vi "LoadMasks.vi"(10 "UiDefinition 2":T1, 11 "ComboBox in":refnum<vi>) -> (0 "error out":errorcluster)   [LabVIEW 2020]
uses:
  UIReferences.ctl
  D:/LabviewDXFViewer/LabviewDXFViewer/bin/Release/LabviewDXFViewer.exe
  LabviewDXFViewer/bin/Release/LabviewDXFViewer.exe
  <vilib>/httpClient/LabVIEWHTTPClient.lvlib
panel:
  out "Array":errorcluster[](array[cluster])
  out "error out 2":errorcluster
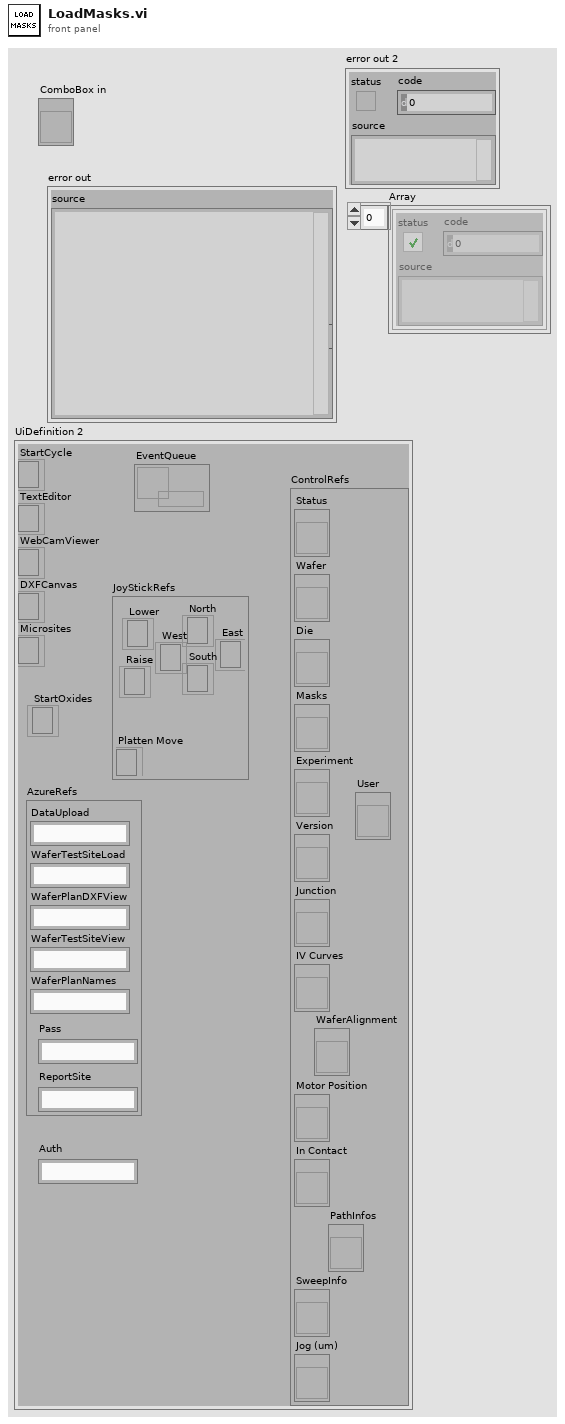
[diagram p1: front panel]
types:
  T1 = typedef "UIReferences.ctl" = cluster{"StartCycle":refnum<k24>, "TextEditor":refnum<k24>, "WebCamViewer":refnum<k24>, "DXFCanvas":refnum<k24>, "Microsites":refnum<k24>, "JoyStickRefs":cluster{"North":refnum<k24>, "Lower":refnum<k24>, "Raise":refnum<k24>, "Platten Move":refnum<k24>, "West":refnum<k24>, "East":refnum<k24>, "South":refnum<k24>}, "AzureRefs":cluster{"DataUpload":string, "WaferTestSiteLoad":string, "WaferPlanDXFView":string, "WaferTestSiteView":string, "WaferPlanNames":string, "Pass":string, "ReportSite":string}, "ControlRefs":cluster{"Status":refnum<vi>, "Wafer":refnum<vi>, "Die":refnum<vi>, "Masks":refnum<vi>, "Experiment":refnum<vi>, "Version":refnum<vi>, "Junction":refnum<vi>, "IV Curves":refnum<vi>, "Motor Position":refnum<vi>, "In Contact":refnum<vi>, "SweepInfo":refnum<vi>, "Jog (um)":refnum<vi>, "PathInfos":refnum<vi>, "User":refnum<vi>, "WaferAlignment":refnum<vi>}, "EventQueue":refnum<queue>, "StartOxides":refnum<k24>, "Auth":string}
  T2 = typedef "LabVIEWHTTPClient.lvlib/ClientHandle.ctl" = refnum<k1>
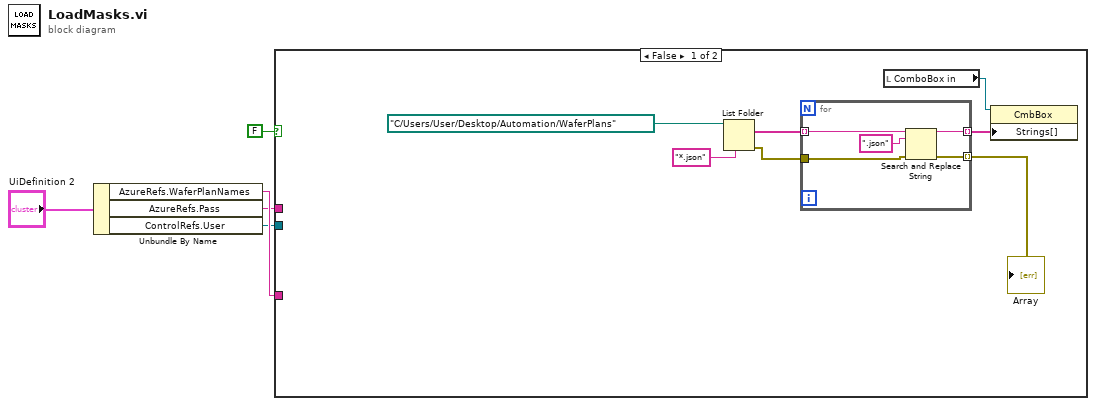
[diagram p0: block diagram]
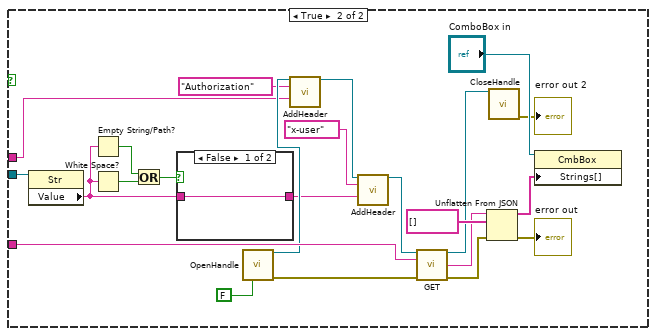
[diagram p2: hidden frame]
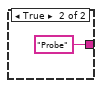
[diagram p3: hidden frame]
diagram:
  n1 = Unbundle By Name("UiDefinition 2") -> ("AzureRefs.WaferPlanNames"=w4:string, "AzureRefs.Pass"=w3:string, "ControlRefs.User"=w2:refnum<vi>)
  n2 = case shown="False" FALSE {
    tunnel: w4 -> [_ w32]
    tunnel: w3 -> [_ w27]
    tunnel: w2 -> [_ w25]
    frame False {
      n3 = List Folder(path=path "C:/Users/User/Desktop/Automation/WaferPlans", pattern="*.json") -> (filenames=w9:string[], error out=w7:errorcluster)  [unwired: 2 in, 2 out]
      n4 = for {
        tunnel: w9 -> [w17] mode=indexing
        tunnel: [w15] -> w8 mode=indexing
        tunnel: w7 -> [w14]
        tunnel: [w13] -> w6 mode=indexing
        n5 = Search and Replace String(input string=w17, search string=".json" ("substring (\"\")"), error in=w14) -> (result string=w15:string, error out=w13:errorcluster)  [unwired: 5 in, 2 out]
      }
      "Array" <- w6
      n6 = local read "ComboBox in"() -> (w11:refnum<vi>)
      n7 = property class="CmbBox"(reference=w11, "Strings[]"=w8) -> ()  [unwired: 1 in, 2 out]
    }
    frame True {
      n8 = property class="Str"(reference=w25) -> ("Value"=w20:string)  [unwired: 1 in, 2 out]
      n9 = Empty String/Path?(string/path=w20) -> (empty?=w21:bool)
      n10 = White Space?(1:w20) -> (0:w24:bool)
      n11 = Or(x=w21, y=w24) -> (x .or. y?=w22:bool)
      n12 = case shown="False" w22 {
        tunnel: w20 -> [w41 _]
        tunnel: [w41 "Probe"] -> w23
        frame False {
        }
        frame True {
        }
      }
      n13 = call <vilib>:"OpenHandle.vi"("verify server(true)"=FALSE) -> ("client handle out"=w31:T2, "error out"=w40:errorcluster)  [unwired: 13 in]
      n14 = call <vilib>:"AddHeader.vi"("client handle"=w31, "header"="Authorization", "value"=w27) -> ("client handle out"=w30:T2)  [unwired: 11 in, 1 out]
      n15 = call <vilib>:"AddHeader.vi"("client handle"=w30, "header"="x-user", "value"=w23) -> ("client handle out"=w29:T2)  [unwired: 11 in, 1 out]
      n16 = call <vilib>:"GET.vi"("client handle"=w29, "url"=w32, "error in (no error)"=w40) -> ("client handle out"=w33:T2, "body"=w34:string, "error out"=w39:errorcluster)  [unwired: 9 in, 1 out]
      n17 = Unflatten From JSON(JSON string=w34, type and defaults=string[] [], error in (no error)=w39) -> (value=w38:string[], error out=→"error out":errorcluster)  [unwired: 4 in]
      n18 = call <vilib>:"CloseHandle.vi"("client handle"=w33) -> ("error out"=→"error out 2":errorcluster)  [unwired: 14 in]
      n19 = property class="CmbBox"(reference="ComboBox in", "Strings[]"=w38) -> ()  [unwired: 1 in, 2 out]
    }
  }
